vi "visa_valve.vi"() -> ()   [LabVIEW 2013]
uses:
  <vilib>/Instr/_visa.llb/VISA Configure Serial Port (Instr).vi
panel:
  out "VISA resource name out":refnum<visa-resource-name>
  out "read buffer":string
  in  "Boolean":bool
  out "error out":errorcluster
  in  "Command option":string
  in  "COMMANDS":T1(ring)
  in  "error in (no error)":errorcluster
  in  "flow control":u16(ring) items=["None"=0, "XON/XOFF"=1, "RTS/CTS"=2, "DTR/DSR"=4]
  in  "stop bits":u16(ring)=10 items=["1.0"=10, "1.5"=15, "2.0"=20]
  in  "parity":u16(ring) items=["None", "Odd", "Even", "Mark", "Space"]
  in  "data bits":u16=8 min=5 max=8 step=1
  in  "VISA resource name":refnum<visa-resource-name>="COM1"
  in  "baud rate":u32=9600
  # "Control Command List\n GO[nn] - Move to nn position \n HM - Move to the first Position \n CW[nn] - Move Clockwise to nn Position \n CC[nn] - Move Counter Clockwise to nn Position \n TO - Toggle Position to Opposite \n TT - Timed Toggle \n DT[nnnnn] - Set Delay time for TT Command \n CP - Returns Current Position \n AM[n] - Sets the Actuator Mode [1] Two Position With Stops, \n [2] Two Position Without Stops, [3] Multi Position \n SB[nnnn] - Set the Baud Rate to nnnnn \n ID[nn] - Set Device ID nn=(0-9, A-Z) \n *ID* - Reset ID to none \n NP[nn] - Set the Number of Positions to nn \n SM[n] - Set the Direction [F]orward, [R]everse, [A]uto \n LRN - Learn Stops Location \n CNT[nnnnn] - Set Cycle Counter \n VR - Firmware Version(s) \n /? - Displays This List"
  # "UNIVERSAL ACTUATOR SETTINGS:\n9600 baud, no parity, 8 data \nbits, 1 stop bit, no hardware or software \nhandshaking."
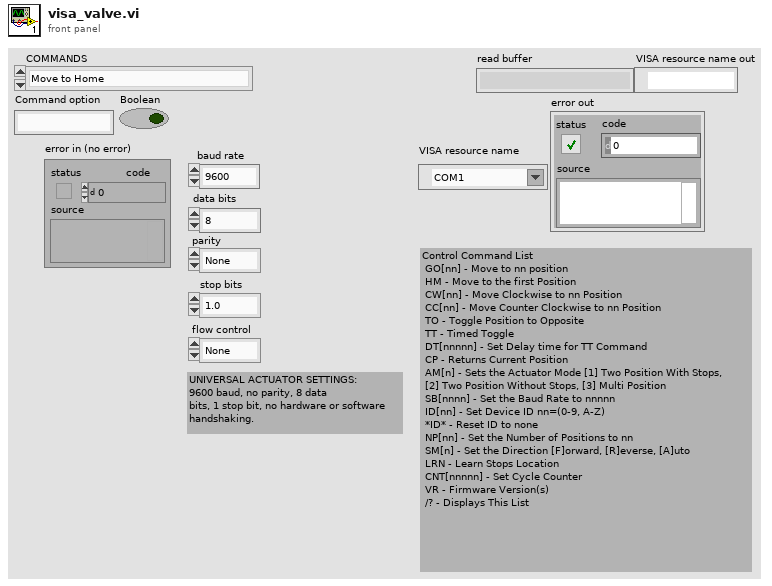
[diagram p1: front panel]
types:
  T1 = enum16{"Move to Home", "Set Positions", "Set Actuator Mode", "OTHER", "Set Direction", "CW Move", "CCW Move"}
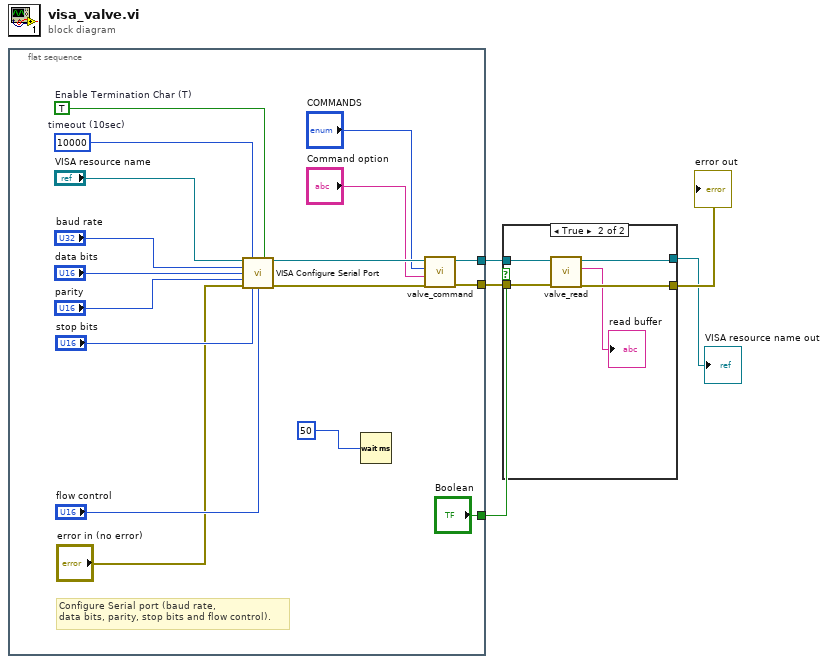
[diagram p0: block diagram]
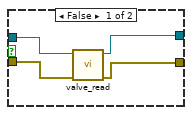
[diagram p2: hidden frame]
diagram:
  n1 = flat-sequence {
    tunnel: [w9] -> w5
    tunnel: [w8] -> w3
    tunnel: ["Boolean"] -> w2
    frame #0 {
      w18 = TRUE  # Enable Termination Char (T)
      w19 = u32 10000  # timeout (10sec)
      # "Configure Serial port (baud rate,\ndata bits, parity, stop bits and flow control)."
      n2 = call-poly "VISA Configure Serial Port"("VISA resource name"="VISA resource name", "timeout (10sec)"=w19, "Enable Termination\nChar (T)"=w18, "baud rate (9600)"="baud rate", "data bits (8)"="data bits", "parity (0:none)"="parity", "error in (no error)"="error in (no error)", "stop bits (10: 1 bit)"="stop bits", "flow control (0:none)"="flow control") -> ("VISA resource name out"=w13:refnum<visa-resource-name>, "error out"=w12:errorcluster)  [unwired: 5 in]
      n3 = Wait (ms)(milliseconds to wait=u32 50) -> ()  [unwired: 1 out]
      n4 = call "valve_command.vi"("Error IN"=w12, "Command option"="Command option", "COMMANDS"="COMMANDS", "VISA Resource IN"=w13) -> ("Error OUT"=w9:errorcluster, "Visa Resource OUT"=w8:refnum<visa-resource-name>)  [unwired: 6 in]
    }
  }
  n5 = case shown="True" w2 {
    tunnel: w5 -> [w25 w31]
    tunnel: [w23 w28] -> w1
    tunnel: [w24 w30] -> w4
    tunnel: w3 -> [w26 w29]
    frame False {
      n6 = call "valve_read.vi"("error in (no error)"=w25, "reference"=w26) -> ("error out"=w24:errorcluster, "VISA resource name out"=w23:refnum<visa-resource-name>)  [unwired: 7 in, 1 out]
    }
    frame True {
      n7 = call "valve_read.vi"("error in (no error)"=w31, "reference"=w29) -> ("error out"=w30:errorcluster, "read buffer"=→"read buffer":string, "VISA resource name out"=w28:refnum<visa-resource-name>)  [unwired: 7 in]
    }
  }
  "error out" <- w4
  "VISA resource name out" <- w1
